vi "DrawBubblePlot.vi"(0 "reference in":refnum<class "LcWebView.lvclass">, 2 "BubblePlot.Dataset":cluster{"x":dbl, "y":dbl, "r":dbl}[][](array[cluster]), 3 "Scatter.DatasetLabels":string[](array[string]), 5 "Error In":errorcluster, 6 "GenericPlotOptions":T1, 7 "BubblePlot.PlotColours":u32[](array[numeric])) -> (14 "reference out":refnum<class "LcWebView.lvclass">, 19 "Error Out":errorcluster)   [LabVIEW 2021, in "LcWebView.lvclass"]
uses:
  LcWebView.lvclass
  ctrls/GenericPlotOption.ctl
  ctrls/LegendPosition.ctl
  cdfa7b6c-348e-4618-b79e-b8b55caa0d01.vi
  <vilib>/JDP Science/JSONtext/Variant to JSON Text.vi
  <vilib>/JDP Science/JSONtext/LVClass Serializer/JSONtext LVClass Serializer.lvclass
  LcWebView.lvclass/LcWebView.ctl
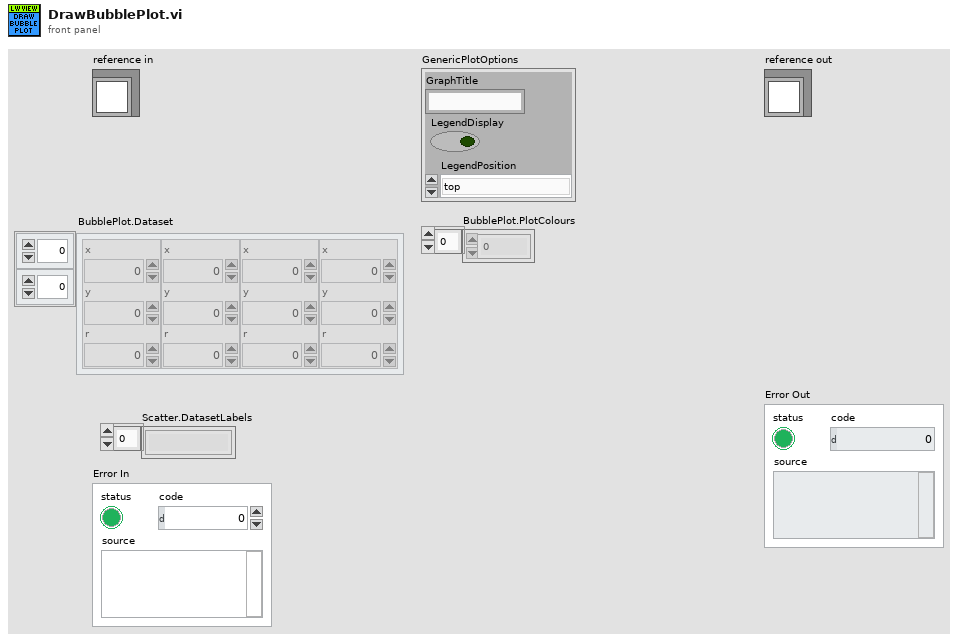
[diagram p1: front panel]
types:
  T1 = typedef "LcWebView.lvclass/GenericPlotOption.ctl" = cluster{"GraphTitle":string, "LegendDisplay":bool, "LegendPosition":T2}
  T2 = typedef "LcWebView.lvclass/LegendPosition.ctl" = enum16{"top", "right", "left", "bottom"}
  T3 = cluster{"action":string, "PlotData":string, "GenericPlotOptions":T1}
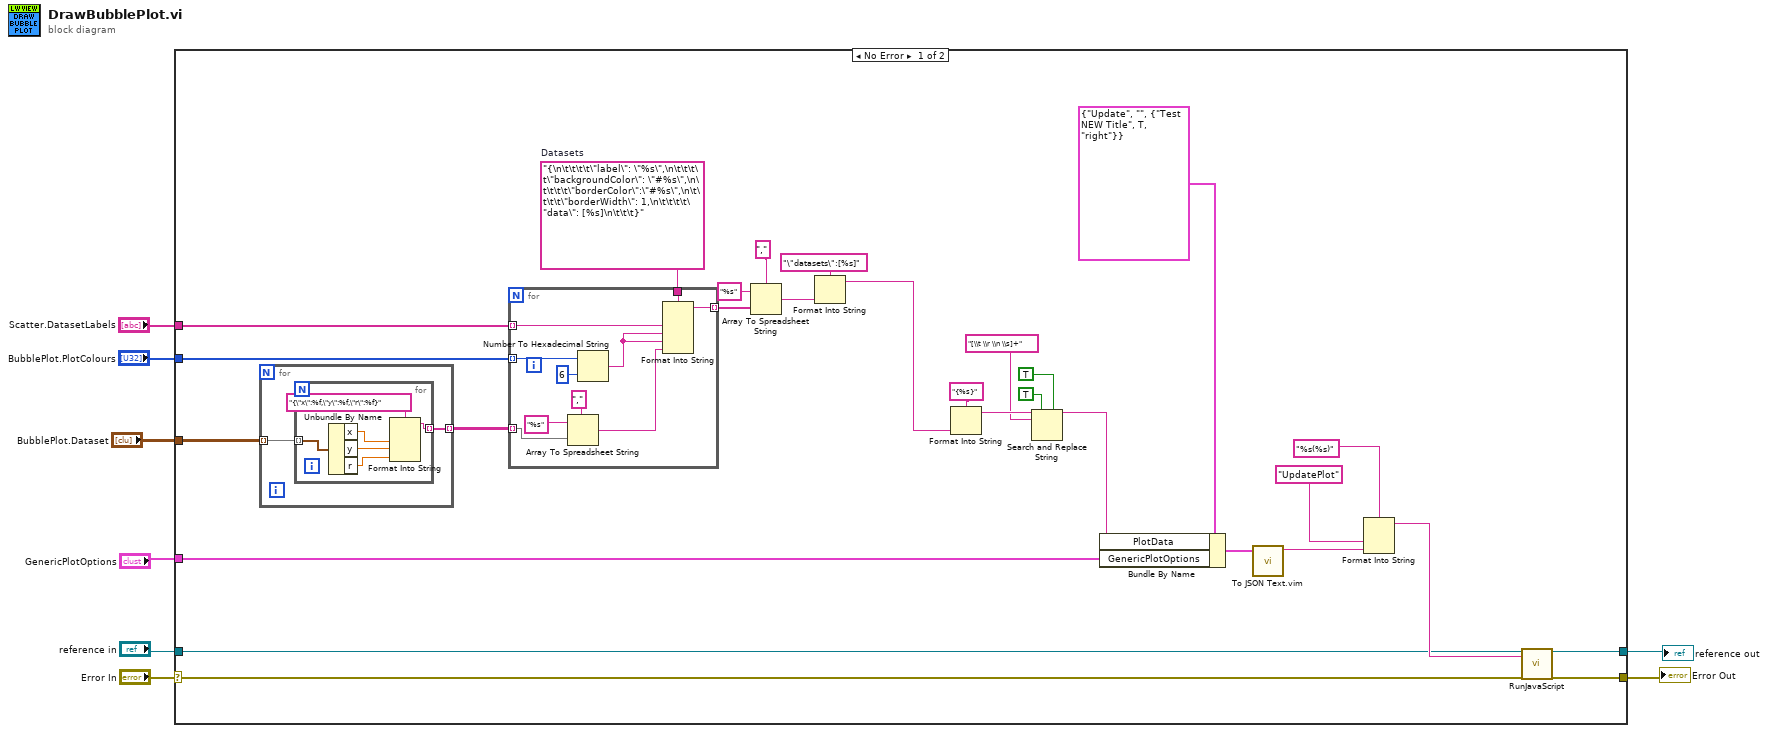
[diagram p0: block diagram]
diagram:
  n1 = case shown="No Error" "Error In" {
    selector: "Error In" -> [w16 w56]
    tunnel: [w17 w56] -> w2
    tunnel: [w18 w55] -> w3
    tunnel: "reference in" -> [w19 w55]
    tunnel: "BubblePlot.Dataset" -> [w11 _]
    tunnel: "BubblePlot.PlotColours" -> [w34 _]
    tunnel: "Scatter.DatasetLabels" -> [w33 _]
    tunnel: "GenericPlotOptions" -> [w26 _]
    frame No Error {
      w35 = "{\n\t\t\t\t\"label\": \"%s\",\n\t\t\t\t\"backgroundColor\": \"#%s\",\n\t\t\t\t\"borderColor\":\"#%s\",\n\t\t\t\t\"borderWidth\": 1,\n\t\t\t\t\"data\": [%s]\n\t\t\t}"  # Datasets
      n2 = for {
        tunnel: w11 -> [w38] mode=indexing
        tunnel: [w37] -> w10 mode=indexing
        n3 = for {
          tunnel: w38 -> [w44] mode=indexing
          tunnel: [w40] -> w37 mode=indexing
          n4 = Unbundle By Name(w44) -> ("x"=w42:dbl, "y"=w41:dbl, "r"=w39:dbl)
          n5 = Format Into String(format string="{\"x\":%f,\"y\":%f,\"r\":%f}", w42, w41, w39) -> (resulting string=w40:string)  [unwired: 2 in, 1 out]
        }
      }
      n6 = for {
        tunnel: w34 -> [w51] mode=indexing
        tunnel: w33 -> [w53] mode=indexing
        tunnel: [w52] -> w15 mode=indexing
        tunnel: w35 -> [w54]
        tunnel: w10 -> [w48] mode=indexing
        n7 = Array To Spreadsheet String(delimiter (Tab)="," ("separator"), array=w48, 3:"%s" ("format string")) -> (spreadsheet string=w45:string)
        n8 = Number To Hexadecimal String(1:i16 6 ("width (-)"), 2:w51) -> (0:w50:string)
        n9 = Format Into String(format string=w54, w53, w50, w50, w45) -> (resulting string=w52:string)  [unwired: 2 in, 1 out]
      }
      n10 = Array To Spreadsheet String(delimiter (Tab)="," ("separator"), array=w15, 3:"%s" ("format string")) -> (spreadsheet string=w12:string)
      n11 = Format Into String(format string="\"datasets\":[%s]", w12) -> (resulting string=w9:string)  [unwired: 2 in, 1 out]
      n12 = Format Into String(format string="{%s}", w9) -> (resulting string=w31:string)  [unwired: 2 in, 1 out]
      n13 = Search and Replace String(replace all?=TRUE ("replace all? (F)"), multiline?=TRUE ("multiline? (F)"), input string=w31, search string="[\\t \\r \\n \\s]+") -> (result string=w30:string)  [unwired: 4 in, 3 out]
      n14 = Bundle By Name(cluster=T3 {"action"="Update", "PlotData"="", "GenericPlotOptions"={"GraphTitle"="Test NEW Title", "LegendDisplay"=TRUE, "LegendPosition"=enum."right"}}, "PlotData"=w30, "GenericPlotOptions"=w26) -> (w24:T3)
      n15 = call "To JSON Text.vim"("Anything"=w24) -> ("<JSON>"=w21:string)  [unwired: 9 in, 1 out]
      n16 = Format Into String(format string="%s(%s)", "UpdatePlot" ("input 1"), w21) -> (resulting string=w20:string)  [unwired: 2 in, 1 out]
      n17 = call-dynamic "RunJavaScript.vi"("reference in"=w19, "Java Script Function"=w20, "Error In"=w16) -> ("reference out"=w18:refnum<class "LcWebView.lvclass">, "Error Out"=w17:errorcluster)  [unwired: 13 in, 2 out]
    }
    frame Error {
    }
  }
  "Error Out" <- w2
  "reference out" <- w3
